vi "Unsubscribe.vi"(8 "error in (no error)":errorcluster, 10 "SubscriptionPolicy":T1, 11 "IObserver in":refnum<class "IObserver.lvclass">) -> (0 "error out":errorcluster, 3 "IObserver out":refnum<class "IObserver.lvclass">)   [LabVIEW 2018, in "MVA Framework.lvlib" / "IObserver.lvlib" / "IObserver.lvclass"]
doc: "取消订阅"
uses:
  IObserver.lvclass
  IMediator/IMediator Messages/Unsubscribe Msg/Unsubscribe Msg.lvclass
  IMediator/ISubscriptionPolicy/ISubscriptionPolicy.lvclass
  IMediator/ISubscriptionPolicy/ISubscriptionPolicy Reference.ctl
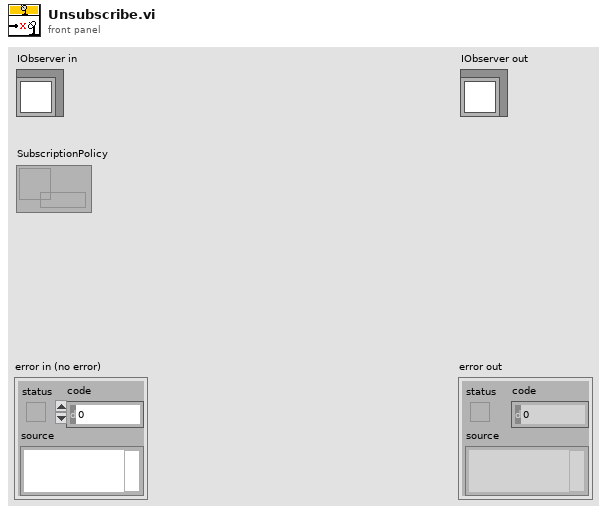
[diagram p1: front panel]
types:
  T1 = typedef "MVA Framework.lvlib/IMediator.lvlib/ISubscriptionPolicy.lvclass/ISubscriptionPolicy Reference.ctl" = refnum<data-value>
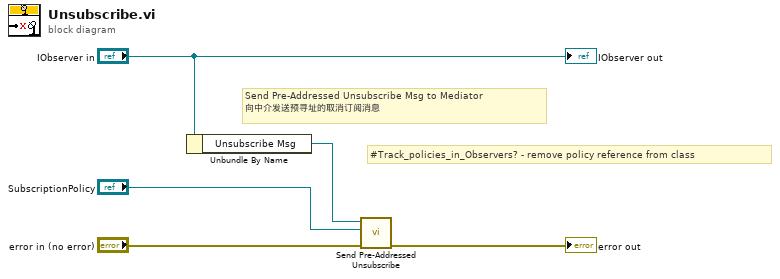
[diagram p0: block diagram]
diagram:
  # "#Track_policies_in_Observers? - remove policy reference from class"
  # "Send Pre-Addressed Unsubscribe Msg to Mediator\n向中介发送预寻址的取消订阅消息"
  n1 = Unbundle By Name("IObserver in") -> ("Unsubscribe Msg"=w4:refnum<class "Unsubscribe Msg.lvclass">)
  n2 = call "Send Pre-Addressed Unsubscribe.vi"("error in (no error)"="error in (no error)", "SubscriptionPolicy"="SubscriptionPolicy", "Unsubscribe Msg In"=w4) -> ("error out"=→"error out":errorcluster)  [unwired: 8 in]
  "IObserver out" <- "IObserver in"
